vi "Class Name.vi"(8 "error in (no error)":errorcluster, 9 "Operation":enum16{"Get", "Set"}(ring), 11 "Class Name":string) -> (0 "error out":errorcluster, 3 "Class Name (out)":string)   [LabVIEW 2017, in "WebServiceImporter.lvlib" / "VI Generator.lvlib"]
uses:
  <vilib>/Platform/WebService/VI Generator/VI Generator.lvlib
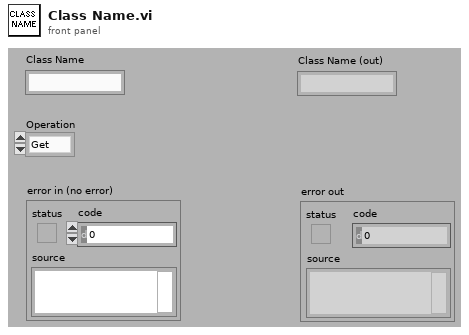
[diagram p1: front panel]
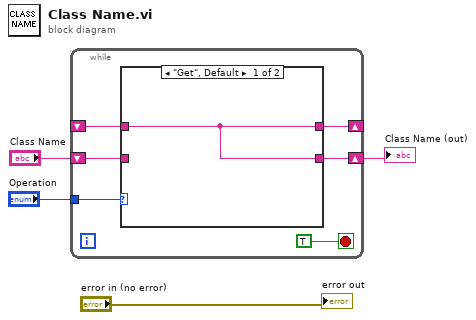
[diagram p0: block diagram]
diagram:
  n1 = while {
    tunnel: "Operation" -> [w10]
    shift-right: [w8] -> w1
    shift-left: "Class Name" -> [w9]
    shift-right: [w7] -> _
    shift-left: _ -> [w6]
    stop <- TRUE stop-if-true
    n2 = case shown="\"Get\", Default" w10 {
      tunnel: w9 -> [_ w12]
      tunnel: [w11 w12] -> w8
      tunnel: [w11 w12] -> w7
      tunnel: w6 -> [w11 _]
      frame "Get", Default {
      }
      frame "Set" {
      }
    }
  }
  "Class Name (out)" <- w1
  "error out" <- "error in (no error)"
